vi "MT Calculate Scaling Factor (PSK).vi"(5 "PSK system parameters":T1 {"PSK type" items=["normal", "shifted", "offset"]; "symbol map" format="%.3f"}, 7 "pulse shaping filter coefficients":dbl[](array[numeric]) format="%.2f", 11 "error in (no error)":errorcluster) -> (6 "waveform scaling factor":dbl, 15 "error out":errorcluster)   [LabVIEW 2020, in "niDMT.lvlib"]
doc: "Calculates the maximum possible waveform amplitude for the PSK modulation scheme."
uses:
  <vilib>/addons/Modulation/niDMT.lvlib
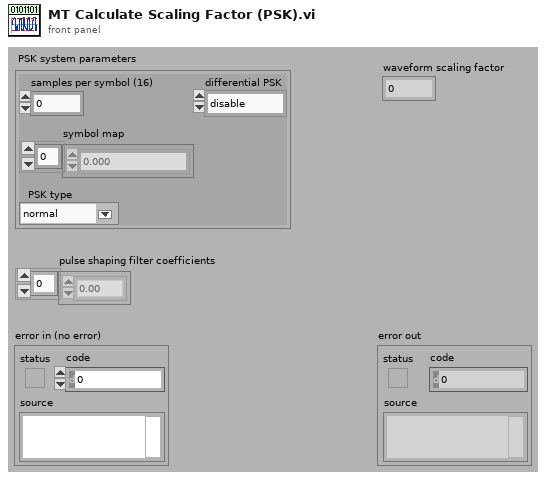
[diagram p1: front panel]
types:
  T1 = cluster{"samples per symbol (16)":i32, "symbol map":cdb[], "differential PSK":enum16{"disable", "enable"}, "PSK type":u16}
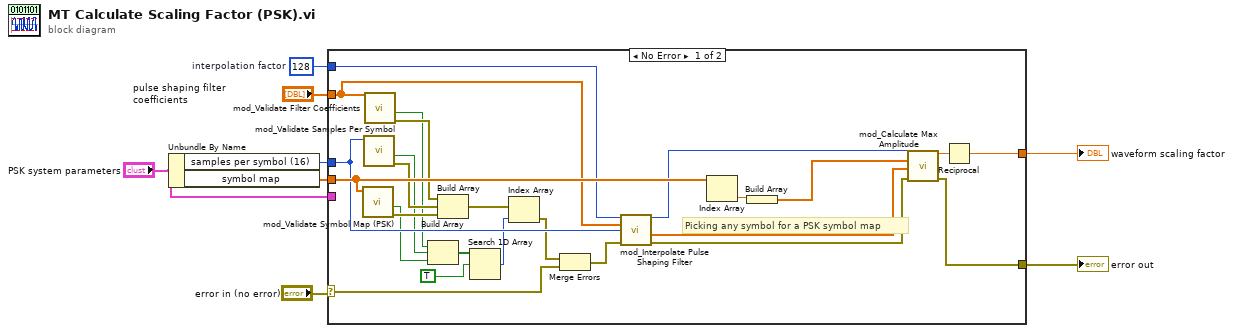
[diagram p0: block diagram]
diagram:
  w8 = 128  # interpolation factor
  n1 = Unbundle By Name("PSK system parameters") -> ("samples per symbol (16)"=w3:i32, "symbol map"=w2:cdb[])
  n2 = case shown="No Error" "error in (no error)" {
    selector: "error in (no error)" -> [w9 w34]
    tunnel: w8 -> [w28 _]
    tunnel: [w32 _] -> w7
    tunnel: "pulse shaping filter coefficients" -> [w27 _]
    tunnel: w3 -> [w26 _]
    tunnel: [w21 w34] -> w4
    tunnel: w2 -> [w29 _]
    tunnel: "PSK system parameters" -> [_ _]
    frame No Error {
      # "Picking any symbol for a PSK symbol map"
      n3 = call <vilib>:"mod_Validate Symbol Map (PSK).vi"("Symbol Map"=w29) -> ("error out"=w18:errorcluster, "error?"=w15:bool)  [unwired: 9 out]
      n4 = call <vilib>:"mod_Validate Samples Per Symbol.vi"("Samples Per Symbol"=w26) -> ("error out"=w19:errorcluster, "error?"=w16:bool)  [unwired: 9 out]
      n5 = call <vilib>:"mod_Validate Filter Coefficients.vi"("Filter Coefficients"=w27) -> ("error out"=w20:errorcluster, "error?"=w17:bool)  [unwired: 9 out]
      n6 = Build Array(w17, w16, w15) -> (w14:bool[])
      n7 = Build Array(w20, w19, w18) -> (w12:errorcluster[])
      n8 = Search 1D Array(1D array=w14, element=TRUE) -> (index of element=w11:i32)  [unwired: 1 out]
      n9 = Index Array(array=w12, index=w11) -> (element=w10:errorcluster)
      n10 = Merge Errors(w10, w9) -> (w23:errorcluster)
      n11 = call <vilib>:"mod_Interpolate Pulse Shaping Filter.vi"("interpolation factor"=w28, "pulse shaping filter coefficients in"=w27, "samples per symbol  in (16 )"=w26, "error in (no error)"=w23) -> ("samples per symbol out (16)"=w25:i32, "pulse shaping filter coefficients out"=w24:dbl[], "error out"=w22:errorcluster)  [unwired: 9 out]
      n12 = Index Array(array=w29) -> (element=w31:cdb)  [unwired: 1 in]
      n13 = Build Array(w31) -> (w30:cdb[])
      n14 = call <vilib>:"mod_Calculate Max Amplitude.vi"("pulse shaping samples per symbol (16)"=w25, "symbol map"=w30, "pulse shaping filter coefficients"=w24, "error in (no error)"=w22) -> ("Max. Amplitude (worst case)"=w33:dbl, "error out"=w21:errorcluster)  [unwired: 10 out]
      n15 = Reciprocal(x=w33) -> (1/x=w32:dbl)
    }
    frame Error {
    }
  }
  "waveform scaling factor" <- w7
  "error out" <- w4
